vi "Hide Panel.vi"(8 "error in (no error)":errorcluster, 11 "View In":refnum<class "View.lvclass">) -> (0 "error out":errorcluster, 3 "View Out":refnum<class "View.lvclass">)   [LabVIEW 2020, in "View.lvclass"]
doc: "Hide the front panel of the View."
uses:
  View.lvclass
  C:/git/astemes-triarc-framework/source/Framework/Process/Process.lvclass
  Process/Process.lvclass/Process.ctl
  Process/Private/SubVIs/Handle Debug Data.vi
  Logging/Log Debug.vi
  <vilib>/AdvancedString/1D String Array to Delimited String.vi
  <vilib>/Utility/High Resolution Relative Seconds.vi
  Process/Public/Read Name.vi
  Callback/Callback.lvclass
  Process/Process.lvclass
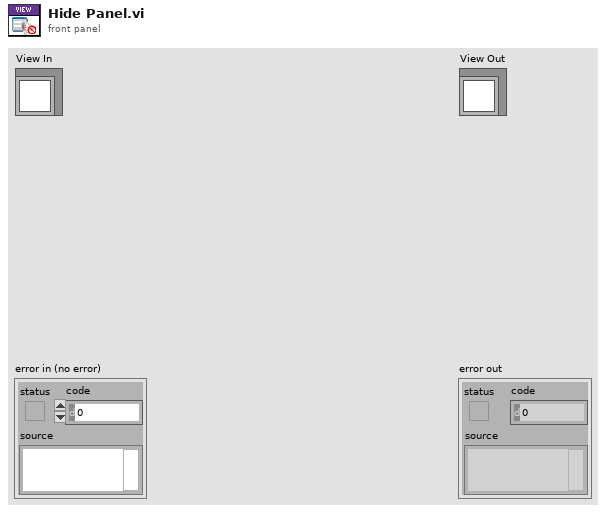
[diagram p1: front panel]
types:
  T1 = typedef "Process.lvclass/API Mode.ctl" = enum16{"Send Message", "Handle Message"}
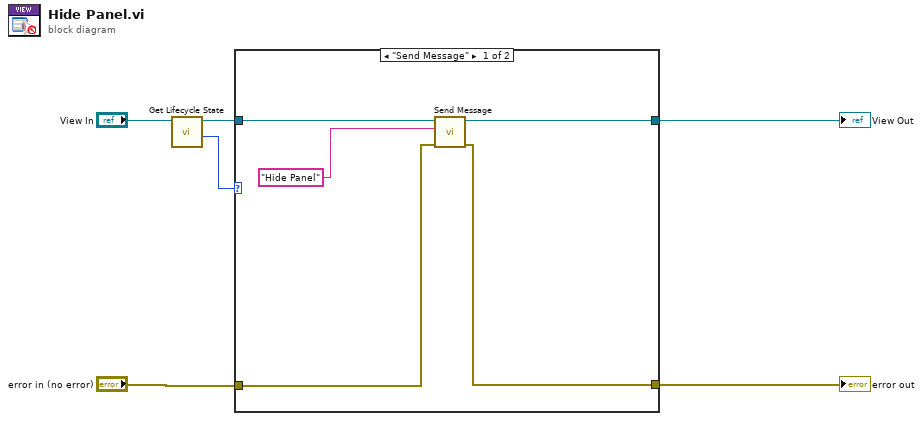
[diagram p0: block diagram]
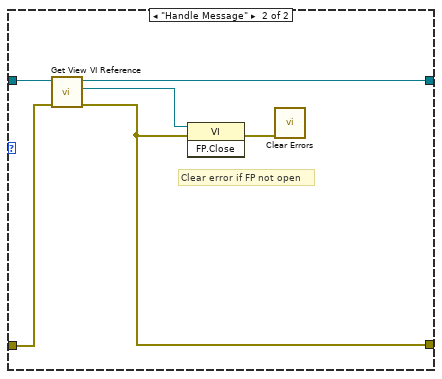
[diagram p2: hidden frame]
diagram:
  n1 = call "Get Lifecycle State.vi"("Process In"="View In") -> ("API Mode"=w2:T1, "Process Out"=w3:refnum<class "View.lvclass">)  [unwired: 7 in, 2 out]
  n2 = case shown="\"Send Message\"" w2 {
    tunnel: [w11 w15] -> w5
    tunnel: [w10 w12] -> w4
    tunnel: "error in (no error)" -> [w9 w14]
    tunnel: w3 -> [w7 w16]
    frame "Send Message" {
      n3 = call "Send Message.vi"("error in (no error)"=w9, "Message"="Hide Panel", "Process In"=w7) -> ("error out"=w10:errorcluster, "Process Out"=w11:refnum<class "View.lvclass">)  [unwired: 7 in]
    }
    frame "Handle Message" {
      # "Clear error if FP not open"
      n4 = call "Get View VI Reference.vi"("error in (no error)"=w14, "View In"=w16) -> ("error out"=w12:errorcluster, "View VI Reference"=w17:refnum<vi>, "View Out"=w15:refnum<class "View.lvclass">)  [unwired: 7 in]
      n5 = invoke class="VI" method="FP.Close"(reference=w17, error in=w12) -> (error out=w13:errorcluster)  [unwired: 1 in, 2 out]
      n6 = call <vilib>:"Clear Errors.vi"("error in (no error)"=w13) -> ()  [unwired: 5 in, 2 out]
    }
  }
  "error out" <- w4
  "View Out" <- w5
